vi "Cxt.vi"() -> ()   [LabVIEW 2010]
uses:
  pulse parameters.ctl
  toolbar icons/log data.ctl
  toolbar icons/Open calibration.ctl
  toolbar icons/Save calibration.ctl
  file/file action.ctl
panel:
  in  "Save Method":T1
  in  "Open Method":T2
  out "signal array":dbl[][](array[numeric])
  out "Save Data":T3
  out "F pulse train graph":cluster{dbl[], dbl[]}[](graph)
  in  "pulse parameters":T4={"Pe"=400.0, "dt"=0.001, "duty"=0.44999999999999996, "cycle time"=0.0, "Integration error"=0.0001, "cycles"=0} {"cycles" min=1; "cycle time" min=0.0; "duty" min=0.0 max=1.0; "dt" min=1e-12; "Pe" min=0.0}
  out "E pulse graph":cluster{"t*":dbl[], dbl[]}(graph)
  in  "stop":bool
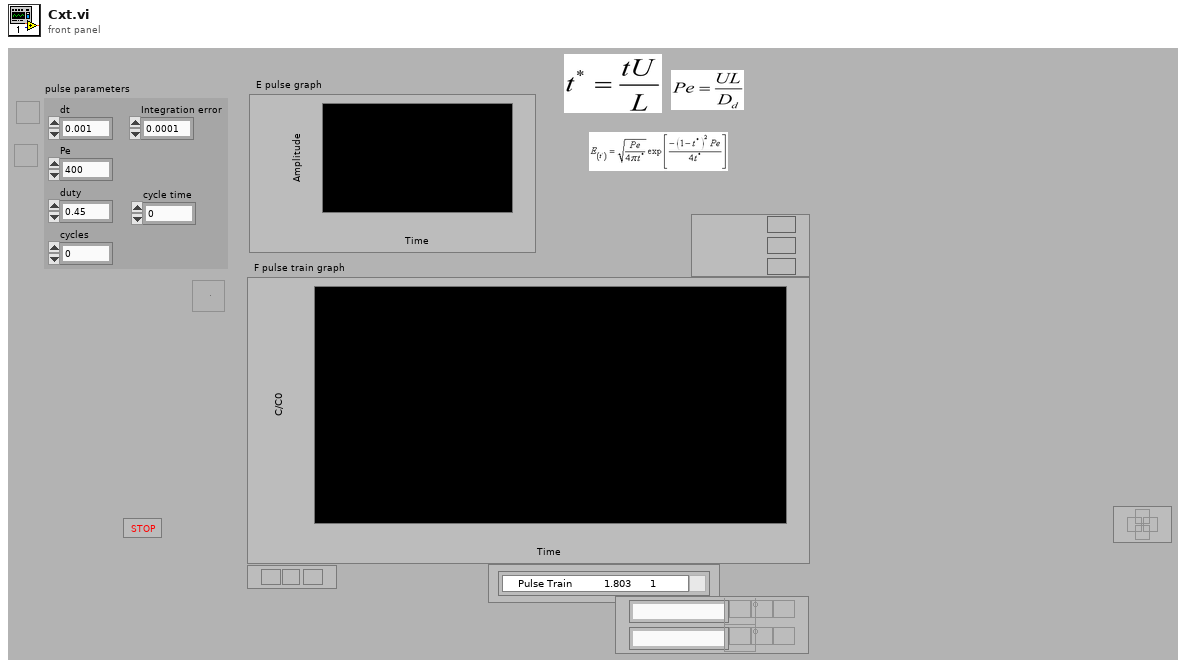
[diagram p1: front panel]
types:
  T1 = typedef "Save calibration.ctl" = bool
  T2 = typedef "Open calibration.ctl" = bool
  T3 = typedef "log data.ctl" = bool
  T4 = typedef "pulse parameters.ctl" = cluster{"Pe":dbl, "dt":dbl, "duty":dbl, "cycle time":dbl, "Integration error":dbl, "cycles":i16}
  T5 = typedef "file action.ctl" = enum16{"Save", "Open"}
  T6 = cluster{"t* pulse train":dbl[], "input waveform":dbl[]}
  T7 = cluster{"Ramp Pattern":dbl[], "input waveform":dbl[]}[]
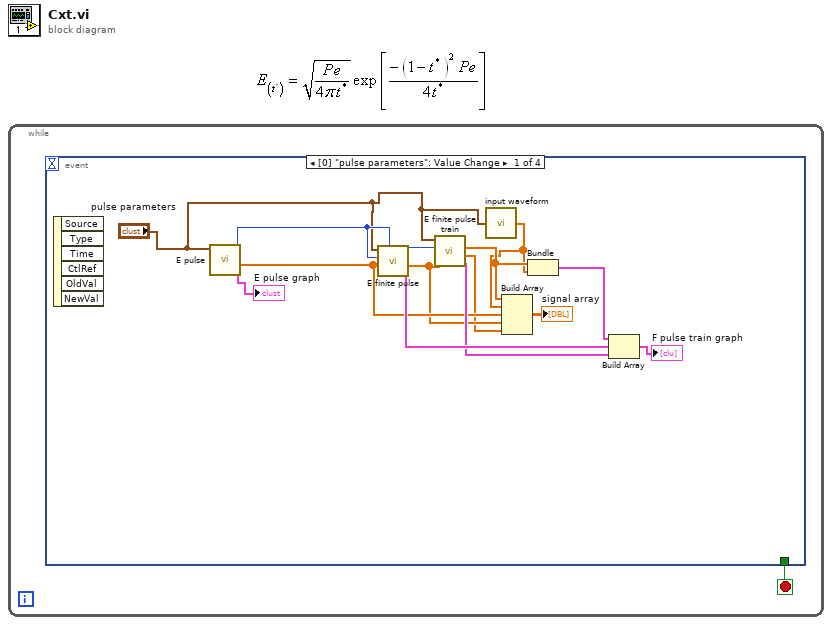
[diagram p0: block diagram]
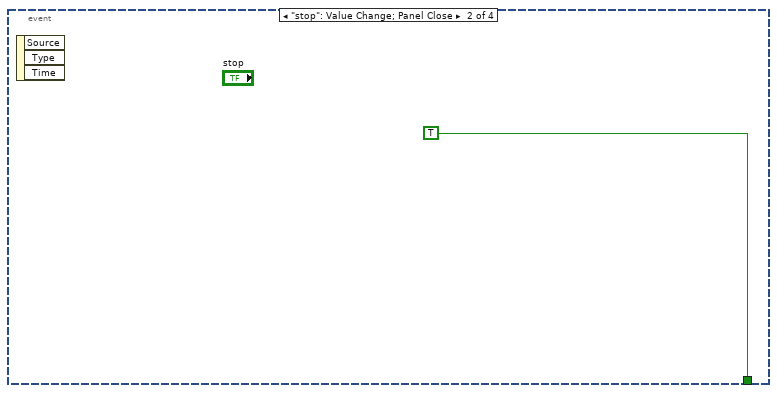
[diagram p2: hidden frame]
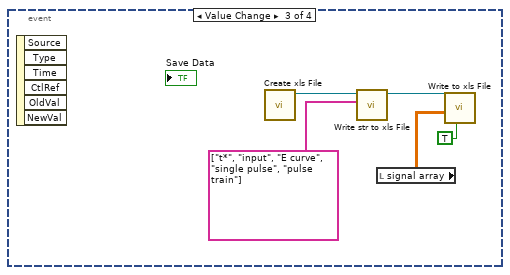
[diagram p3: hidden frame]
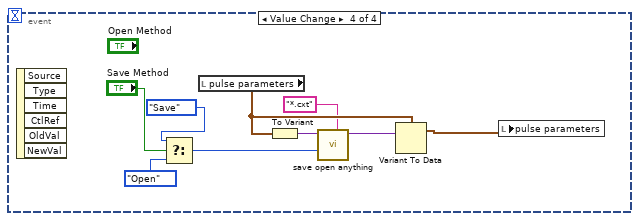
[diagram p4: hidden frame]
diagram:
  n1 = while {
    stop <- w1 stop-if-true
    n2 = event shown="[0] \"pulse parameters\": Value Change" {
      selector: _ -> [_ _ _ _]
      dyn-events: _ -> [_ _ _ _]
      timeout: _ -> [_ _ _ _]
      tunnel: [_ TRUE _ _] -> w1
      event Value Change {
        n3 = event-data() -> ()  [unwired: 1 in, 6 out]
        n4 = call "E pulse.vi"("pulse parameters"="pulse parameters") -> ("E graph"=→"E pulse graph":cluster{"t*":dbl[], dbl[]}, "E"=w5:dbl[], "t*/theta"=w14:i16)  [unwired: 7 in, 1 out]
        n5 = call "E finite pulse.vi"("E"=w5, "t*/theta"=w14, "pulse parameters"="pulse parameters") -> ("F finite graph"=w12:cluster{"t*":dbl[], dbl[]}, "F finite"=w4:dbl[])  [unwired: 6 in, 1 out]
        n6 = call "E finite pulse train.vi"("F finite"=w4, "t*/theta"=w14, "pulse parameters"="pulse parameters") -> ("F pulse train graph"=w11:cluster{"Ramp Pattern":dbl[], dbl[]}, "F pulse train"=w3:dbl[], "t* pulse train"=w7:dbl[])  [unwired: 6 in]
        n7 = call "input waveform.vi"("pulse parameters"="pulse parameters") -> ("input waveform"=w6:dbl[])
        n8 = Build Array(w7, w6, w5, w4, w3) -> (→"signal array":dbl[][])
        n9 = Bundle("t* pulse train"=w7, "input waveform"=w6) -> (w8:T6)  [unwired: 1 in]
        n10 = Build Array(w8, w12, w11) -> (→"F pulse train graph":T7)
      }
      event "stop": Value Change; Panel Close {
        n11 = event-data() -> ()  [unwired: 1 in, 3 out]
      }
      event Value Change {
        n12 = event-data() -> ()  [unwired: 1 in, 6 out]
        n13 = call "Create xls File.vi"() -> ("refnum"=w20:refnum<file>)  [unwired: 4 in, 3 out]
        n14 = call "Write str to xls File.vi"("1D data"=string[] ["t*", "input", "E curve", "single pulse", "pulse train"], "refnum"=w20) -> ("dup refnum"=w19:refnum<file>)  [unwired: 8 in, 1 out]
        n15 = local read "signal array"() -> (w17:dbl[][])
        n16 = call "Write to xls File.vi"("transpose? (no:F)"=TRUE, "2D data"=w17, "refnum"=w19) -> ()  [unwired: 7 in, 2 out]
      }
      event Value Change {
        n17 = event-data() -> ()  [unwired: 1 in, 6 out]
        n18 = Select(t=file_action."Save" ("Action"), s="Save Method", f=file_action."Open" ("Action")) -> (s? t:f=w26:T5)
        n19 = local read "pulse parameters"() -> (w23:T4)
        n20 = To Variant(anything=w23) -> (Variant=w29:variant)
        n21 = call "save open anything.vi"("Variant"=w29, "Action"=w26, "pattern"="*.cxt") -> ("Variant out"=w24:variant)  [unwired: 4 in, 3 out]
        n22 = Variant To Data(Variant=w24, type=w23) -> (data=w22:T4)  [unwired: 1 in, 1 out]
        n23 = local write "pulse parameters"(w22) -> ()
      }
    }
  }
